vi "DHE_RunProc.vi"(7 "VItoRun":string, 11 "error in (no error)":errorcluster, 12 "wait":bool=TRUE) -> (6 "Result":string, 8 "wait imdone":bool, 15 "error out":errorcluster)   [LabVIEW 2016]
uses:
  <vilib>/Utility/error.llb/DialogType.ctl
panel:
  in  "type specifier VI Refnum (for type only)":refnum<vi>
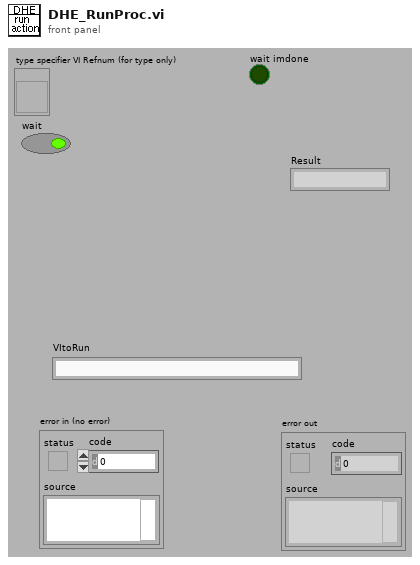
[diagram p1: front panel]
types:
  T1 = enum16{"Idle", "Exposing", "Paused", "AbortExp", "Reading", "AbortRead", "FinishedReading", "Resetting", "Reducing", "Initializing"}
  T2 = cluster{"Video Processor Type":string, "support gain":bool, "Timing Board":string, "support reset":bool, "Utility Board":string, "Shutter":string, "Temperature":string, "support temp control":bool, "Detector Type":string, "Support MPP":string, "Support Binning":string, "Readout Mode":string, "support shutter control":bool}
  T3 = typedef "DialogType.ctl" = u16
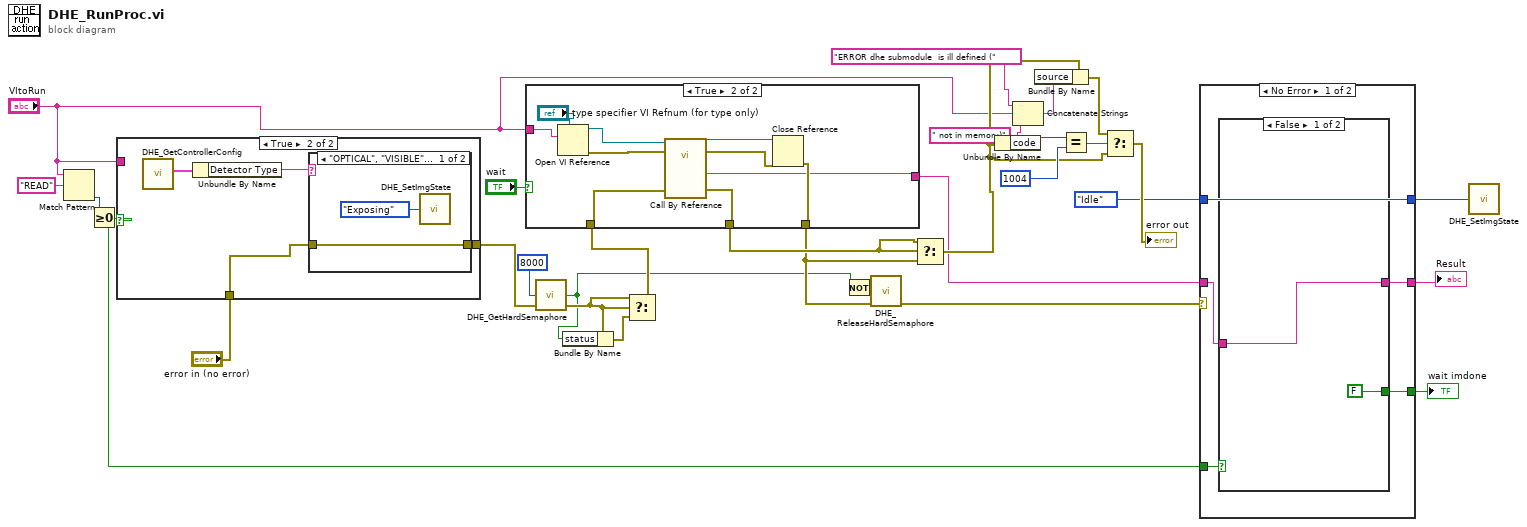
[diagram p0: block diagram]
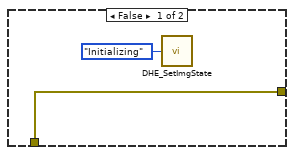
[diagram p2: hidden frame]
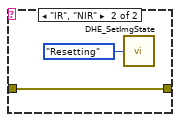
[diagram p3: hidden frame]
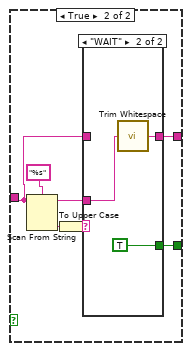
[diagram p4: hidden frame]
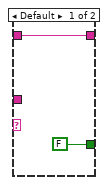
[diagram p5: hidden frame]
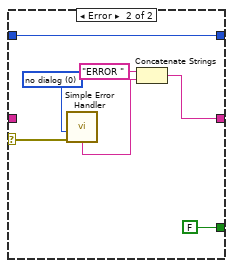
[diagram p6: hidden frame]
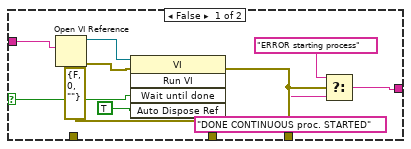
[diagram p7: hidden frame]
diagram:
  n1 = Match Pattern(string="VItoRun", regular expression="READ") -> (offset past match=w19:i32)  [unwired: 4 out]
  n2 = Greater Or Equal To 0?(x=w19) -> (x >= 0?=w6:bool)
  n3 = case shown="True" w6 {
    tunnel: [w32 w36] -> w17
    tunnel: "error in (no error)" -> [w32 w33]
    tunnel: "VItoRun" -> [_ _]
    frame False {
      n4 = call "DHE_SetImgState.vi"("DHE_ImgState"=T1."Initializing") -> ()  [unwired: 9 out]
    }
    frame True {
      n5 = call "DHE_GetControllerConfig.vi"() -> ("ControllerConfigCluster"=w35:T2)  [unwired: 11 out]
      n6 = Unbundle By Name(w35) -> ("Detector Type"=w34:string)
      n7 = case shown="\"OPTICAL\", \"VISIBLE\", Default" w34 {
        tunnel: w33 -> [w38 w40]
        tunnel: [w38 w40] -> w36
        frame "OPTICAL", "VISIBLE", Default {
          n8 = call "DHE_SetImgState.vi"("DHE_ImgState"=T1."Exposing") -> ()  [unwired: 9 out]
        }
        frame "IR", "NIR" {
          n9 = call "DHE_SetImgState.vi"("DHE_ImgState"=T1."Resetting") -> ()  [unwired: 9 out]
        }
      }
    }
  }
  n10 = call "DHE_GetHardSemaphore.vi"("timeout"=8000, "error in (no error)"=w17) -> ("timed out"=w10:bool, "error out"=w12:errorcluster)  [unwired: 6 out]
  n11 = Bundle By Name(cluster=w12, "status"=w10) -> (w11:errorcluster)
  n12 = Select(t=w12, s=w12, f=w11) -> (s? t:f=w13:errorcluster)
  n13 = case shown="True" "wait" {
    selector: "wait" -> [w50 _]
    tunnel: [w48 w60] -> w15
    tunnel: w13 -> [_ w51]
    tunnel: [errorcluster {"status"=FALSE, "code"=0, "source"=""} ("error out") w59] -> w23
    tunnel: [w45 w56] -> w22
    tunnel: "VItoRun" -> [w44 w52]
    frame False {
      n14 = Open VI Reference(vi path=w44) -> (vi reference=w43:refnum<vi>, error out=w42:errorcluster)  [unwired: 2 in, 3 out]
      n15 = invoke class="VI" method="Run VI"(reference=w43, error in=w42, "Wait until done"=w50, "Auto Dispose Ref"=TRUE ("Auto Dispose Reference")) -> (error out=w48:errorcluster)  [unwired: 1 in, 4 out]
      n16 = Select(t="ERROR starting process", s=w48, f="DONE CONTINUOUS proc. STARTED" ("Message")) -> (s? t:f=w45:string)
    }
    frame True {
      n17 = Open VI Reference(type specifier VI Refnum (for type only)="type specifier VI Refnum (for type only)", vi path=w52) -> (vi reference=w54:refnum<vi>, error out=w55:errorcluster)  [unwired: 2 in, 2 out]
      n18 = call-by-ref "?"(reference=w54, error in=w55, "error in"=w51) -> (reference out=w57:refnum<vi>, error out=w58:errorcluster, 0:"error out"=w59:errorcluster, "response"=w56:string)  [unwired: 9 in]
      n19 = Close Reference(reference=w57, error in (no error)=w58) -> (error out=w60:errorcluster)
    }
  }
  n20 = Not(x=w10) -> (.not. x?=w9:bool)
  n21 = call "DHE_ReleaseHardSemaphore.vi"("error in (no error)"=w15, "release?"=w9) -> ("error out"=w14:errorcluster)  [unwired: 9 out]
  n22 = Select(t=w23, s=w23, f=w15) -> (s? t:f=w27:errorcluster)
  n23 = Unbundle By Name(w27) -> ("code"=w30:i32)
  n24 = Concatenate Strings("ERROR dhe submodule  is ill defined (" ("source"), "VItoRun", " not in memory)") -> (w2:string)
  n25 = Bundle By Name(cluster=w27, "source"=w2) -> (w26:errorcluster)
  n26 = Equal?(x=w30, y=1004) -> (x = y?=w28:bool)
  n27 = Select(t=w26, s=w28, f=w27) -> (s? t:f=→"error out":errorcluster)
  n28 = case shown="No Error" w14 {
    selector: w14 -> [_ w86]
    tunnel: w22 -> [w62 _]
    tunnel: [w61 w80] -> w21
    tunnel: T1."Idle" ("DHE_ImgState") -> [w65 w84]
    tunnel: [w65 w84] -> w7
    tunnel: w6 -> [w64 _]
    tunnel: [w63 FALSE] -> w5
    frame No Error {
      n29 = case shown="False" w64 {
        tunnel: w62 -> [w66 w68]
        tunnel: [FALSE w69] -> w63
        tunnel: [w66 w70] -> w61
        frame False {
        }
        frame True {
          n30 = Scan From String(format string="%s", input string=w68) -> (remaining string=w71:string, output 1=w73:string)  [unwired: 2 in, 3 out]
          n31 = To Upper Case(1:w73) -> (0:w72:string)
          n32 = case shown="\"WAIT\"" w72 {
            tunnel: w71 -> [_ w79]
            tunnel: [w76 w78] -> w70
            tunnel: [FALSE TRUE] -> w69
            tunnel: w68 -> [w76 _]
            frame Default {
            }
            frame "WAIT" {
              n33 = call <vilib>:"Trim Whitespace.vi"("string"=w79) -> ("trimmed string"=w78:string)  [unwired: 1 in]
            }
          }
        }
      }
    }
    frame Error {
      w85 = T3 0 items=["no dialog", "OK message", "continue or stop message", "OK message + warnings", "continue/stop + warnings"] ("type of dialog (OK msg:1)")
      n34 = call <vilib>:"Simple Error Handler.vi"("type of dialog (OK msg:1)"=w85, "error in (no error)"=w86) -> ("message"=w81:string)  [unwired: 7 out]
      n35 = Concatenate Strings("ERROR " ("string"), w81) -> (w80:string)
    }
  }
  "Result" <- w21
  "wait imdone" <- w5
  n36 = call "DHE_SetImgState.vi"("DHE_ImgState"=w7) -> ()  [unwired: 9 out]
